vi "IAmGLF-DeleteDVR.vi"(8 "error in (no error)":errorcluster, 11 "Engine in":refnum<class "Engine.lvclass">) -> (0 "error out":errorcluster, 3 "Engine out":refnum<class "Engine.lvclass">)   [LabVIEW 2024, in "GLF.lvlib" / "Engine.lvclass"]
doc: "<B>Summary</B>\nTo delete the class DVR from standalone process."
uses:
  Engine.lvclass
  Engine.lvclass/Engine.ctl
  IAmGLF/IAmGLF.lvclass
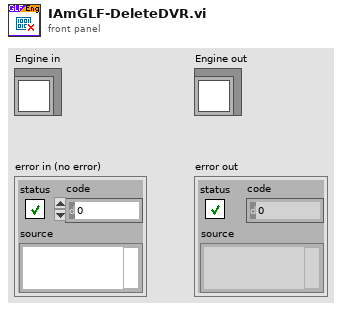
[diagram p1: front panel]
types:
  T1 = typedef "GLF.lvlib/Engine.lvclass/DVR--cluster.ctl" = cluster{"CMD Queue":T2, "Config":T3, "Ctxt":T5, "Metrics":T6, "GLF Instances":refnum<class "IAmGLF.lvclass">[]}
  T2 = typedef "GLF.lvlib/Engine.lvclass/Command--queue.ctl" = refnum<queue>
  T3 = typedef "GLF.lvlib/Engine.lvclass/Config--cluster.ctl" = cluster{"Quit On Last Window Closed":bool, "VSync":T4, "FPS Target":dbl}
  T4 = typedef "GLF.lvlib/Engine.lvclass/VSync--enum.ctl" = enum16{"Disabled", "Enabled", "Adaptative"}
  T5 = typedef "GLF.lvlib/Engine.lvclass/Context--cluster.ctl" = cluster{"Ticks Begin":u64, "VSync Enabled":bool}
  T6 = typedef "GLF.lvlib/Engine.lvclass/Metrics--cluster.ctl" = cluster{"Uptime [ms]":u64, "Loop Time [ms]":u64}
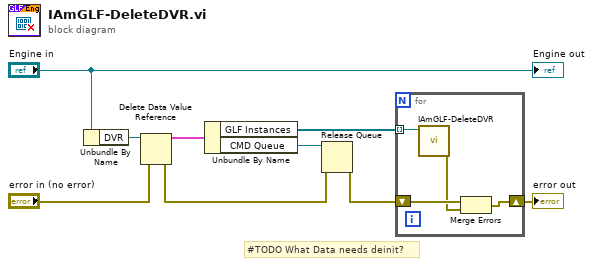
[diagram p0: block diagram]
diagram:
  # "#TODO What Data needs deinit?"
  n1 = Unbundle By Name("Engine in") -> ("DVR"=w9:refnum<data-value>)
  n2 = Delete Data Value Reference(data value reference=w9, error in="error in (no error)") -> (data value=w8:T1, error out=w4:errorcluster)
  n3 = Unbundle By Name(w8) -> ("GLF Instances"=w3:refnum<class "IAmGLF.lvclass">[], "CMD Queue"=w7:T2)
  n4 = Release Queue(queue=w7, error in (no error)=w4) -> (error out=w2:errorcluster)  [unwired: 1 in, 2 out]
  n5 = for {
    tunnel: w3 -> [w13] mode=indexing
    shift-right: [w11] -> w1
    shift-left: w2 -> [w12]
    n6 = call-dynamic "IAmGLF-DeleteDVR.vi"("IAmGLF in"=w13) -> ("error out"=w10:errorcluster)  [unwired: 9 in, 1 out]
    n7 = Merge Errors(w12, w10) -> (w11:errorcluster)
  }
  "error out" <- w1
  "Engine out" <- "Engine in"
